vi "Create TLS Config.vi"(11 "TLS Config":T1) -> (0 "error out":errorcluster, 3 "Immutable TLS":refnum<k36>, 5 "TLS Enabled":bool)   [LabVIEW 2020, in "TCP Comms.lvlib"]
uses:
  TCP Comms.lvlib
  Cert Chain.ctl
  TLS Config.ctl
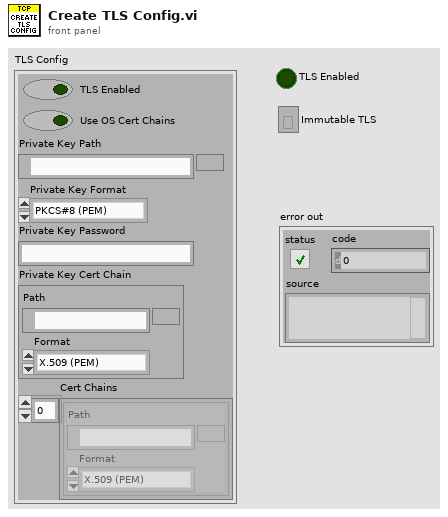
[diagram p1: front panel]
types:
  T1 = typedef "TCP Comms.lvlib/TLS Config.ctl" = cluster{"TLS Enabled":bool, "Use OS Cert Chains":bool, "Private Key Path":path, "Private Key Format":enum32{"PKCS#8 (PEM)", "PKCS#8 (DER)"}, "Private Key Password":string, "Private Key Cert Chain":T2, "Cert Chains":T2[]}
  T2 = typedef "TCP Comms.lvlib/Cert Chain.ctl" = cluster{"Path":path, "Format":enum32{"X.509 (PEM)"}}
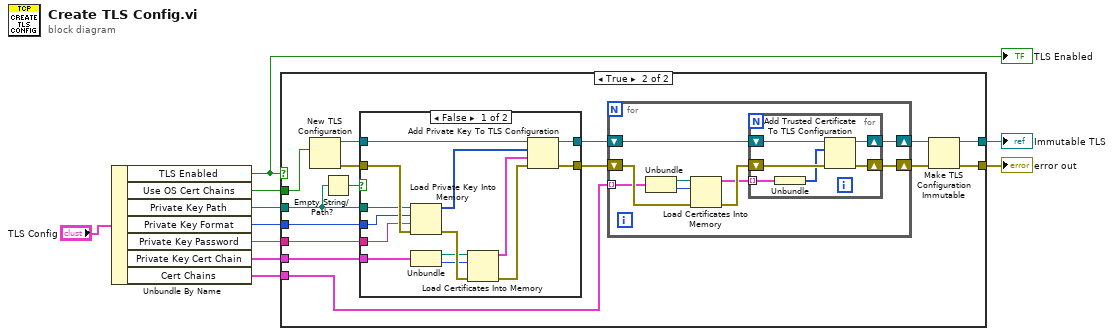
[diagram p0: block diagram]
diagram:
  n1 = Unbundle By Name("TLS Config") -> ("TLS Enabled"=w9:bool, "Use OS Cert Chains"=w8:bool, "Private Key Path"=w7:path, "Private Key Format"=w6:enum32{"PKCS#8 (PEM)", "PKCS#8 (DER)"}, "Private Key Password"=w5:string, "Private Key Cert Chain"=w4:T2, "Cert Chains"=w1:T2[])
  "TLS Enabled" <- w9
  n2 = case shown="True" w9 {
    tunnel: w8 -> [_ w25]
    tunnel: w7 -> [_ w21]
    tunnel: w6 -> [_ w20]
    tunnel: w5 -> [_ w19]
    tunnel: w4 -> [_ w18]
    tunnel: [_ w13] -> w3
    tunnel: [_ w12] -> w2
    tunnel: w1 -> [_ w11]
    frame False {
    }
    frame True {
      n3 = New TLS Configuration(10:w25) -> (0:w22:errorcluster, 3:w23:refnum<k36>)  [unwired: 1 in]
      n4 = Empty String/Path?(string/path=w21) -> (empty?=w24:bool)
      n5 = case shown="False" w24 {
        tunnel: w23 -> [w49 w56]
        tunnel: w22 -> [w53 w55]
        tunnel: w21 -> [w52 _]
        tunnel: w20 -> [w51 _]
        tunnel: [w46 w56] -> w17
        tunnel: [w47 w55] -> w16
        tunnel: w19 -> [w50 _]
        tunnel: w18 -> [w45 _]
        frame False {
          n6 = Load Private Key Into Memory(8:w53, 9:w50, 10:w51, 11:w52) -> (0:w54:errorcluster, 3:w48:u8[])
          n7 = Unbundle(w45) -> ("Path"=w44:path, "Format"=w43:enum32{"X.509 (PEM)"})
          n8 = Load Certificates Into Memory(8:w54, 10:w43, 11:w44) -> (0:w41:errorcluster, 3:w42:cluster{"certificate":u8[]}[])
          n9 = Add Private Key To TLS Configuration(8:w41, 9:w42, 10:w48, 11:w49) -> (0:w47:errorcluster, 3:w46:refnum<k36>)
        }
        frame True {
        }
      }
      n10 = for {
        shift-right: [w27] -> w15
        shift-left: w17 -> [w29]
        shift-right: [w26] -> w14
        shift-left: w16 -> [w33]
        tunnel: w11 -> [w32] mode=indexing
        n11 = Unbundle(w32) -> ("Path"=w31:path, "Format"=w30:enum32{"X.509 (PEM)"})
        n12 = Load Certificates Into Memory(8:w33, 10:w30, 11:w31) -> (0:w34:errorcluster, 3:w28:cluster{"certificate":u8[]}[])
        n13 = for {
          shift-right: [w39] -> w27
          shift-left: w29 -> [w40]
          tunnel: w28 -> [w36] mode=indexing
          shift-right: [w37] -> w26
          shift-left: w34 -> [w38]
          n14 = Unbundle(w36) -> ("certificate"=w35:u8[])
          n15 = Add Trusted Certificate To TLS Configuration(8:w38, 10:w35, 11:w40) -> (0:w37:errorcluster, 3:w39:refnum<k36>)
        }
      }
      n16 = Make TLS Configuration Immutable(8:w14, 11:w15) -> (0:w12:errorcluster, 3:w13:refnum<k36>)
    }
  }
  "Immutable TLS" <- w3
  "error out" <- w2
